vi "Read supported data types.vi"(8 "error in":errorcluster, 11 "DecideProjectFeatures in":refnum<class "TagBusConfigurablePluginDecideFeatures.lvclass">) -> (0 "error out":errorcluster, 2 "supported data types":T1[](array[typedef]), 3 "DecideProjectFeatures out":refnum<class "TagBusConfigurablePluginDecideFeatures.lvclass">)   [LabVIEW 2013, in "TagBusConfigurablePluginDecideFeatures.lvclass"]
uses:
  TagBusConfigurablePluginDecideFeatures.lvclass
  <vilib>/NI/Tag Bus/tag/Data Type.ctl
  TagBusConfigurablePluginDecideFeatures.lvclass/TagBusConfigurablePluginDecideFeatures.ctl
  <vilib>/NI/Tag Bus/tag/tag descriptor.lvclass
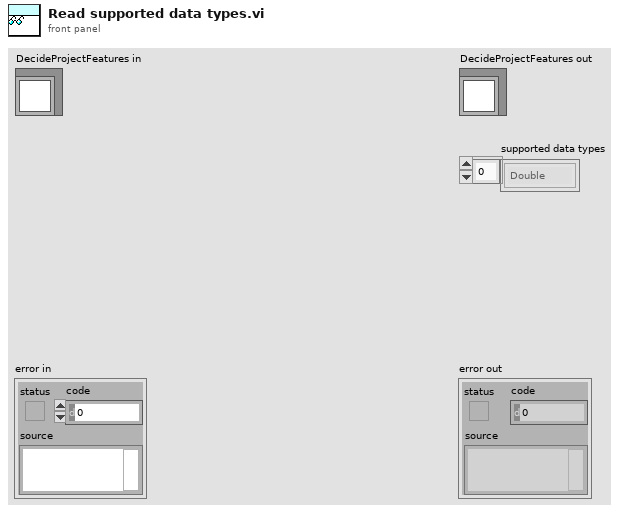
[diagram p1: front panel]
types:
  T1 = typedef "tag bus.lvlib/tag descriptor.lvclass/Data Type.ctl" = enum16{"Double", "Single", "I64", "I32", "I16", "I8", "U64", "U32", "U16", "U8", "Boolean", "String", "Array of Double", "Array of Single", "Array of I64", "Array of I32", "Array of I16", "Array of I8", "Array of U64", "Array of U32", "Array of U16", "Array of U8", "Array of Boolean", "Array of String"}
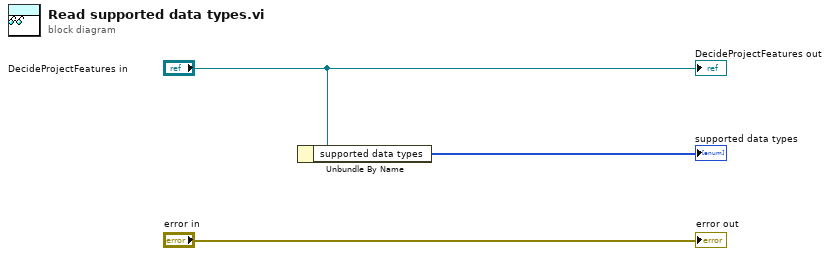
[diagram p0: block diagram]
diagram:
  n1 = Unbundle By Name("DecideProjectFeatures in") -> ("supported data types"=→"supported data types":T1[])
  "error out" <- "error in"
  "DecideProjectFeatures out" <- "DecideProjectFeatures in"
